vi "Query Instrument Version.vi"(0 "VISA resource name":refnum<visa-resource-name>, 5 "FPGA (0:Hardware Controller FPGA on Main Unit)":i32(ring) items=["Hardware Controller FPGA on Main Unit", "Control PLD And Panel on Main Unit", "Measure PCI FPGA on Main Unit", "Measure Core FPGA on Main Unit", "Measure COM DSP on Main Unit", "RF FPGA on SA RF Unit", "RF FPGA on SA 13GHz RF Unit", "Baseband FPGA on VSG Unit", "RF FPGA on VSG Unit", "Down Conv FPGA on Down Convertor Unit", "2nd Conv FPGA on 2nd Convertor Unit", "ATT_Driver FPGA on ATT Driver Unit", "Hardware Controller FPGA", "Control PLD And Panel", "IF/Local FPGA", "RF/Micro FPGA", "PCI FPGA on Measure Unit", "Core FPGA on Measure Unit", "COM DSP on Measure Unit", "Core FPGA on Measure Option Unit", "Baseband FPGA on SG Unit", "RF FPGA on SG Unit", "BBIF Interface FPGA", "BBIF Main FPGA", "BBIF PCI FPGA", "All FPGA"], 7 "Application (0:Signal Analyzer)":i32(ring) items=["Signal Analyzer", "Spectrum Analyzer", "Phase Noise", "Power Meter", "BER Test"], 9 "Hardware (0:Main Unit)":i32(ring) items=["Main Unit", "SA RF Unit", "SA 13GHz RF Unit", "VSG Unit", "Down Converter Unit", "2nd Converter Unit", "ATT_Driver Unit", "Revision number", "IF Unit", "IF/Local Unit", "RF/Micro Unit", "Measure Unit", "Measure Option Unit", "SG Unit", "CPU Unit", "BBIF Unit", "All"], 11 "error in (no error)":errorcluster) -> (4 "VISA resource name out":refnum<visa-resource-name>, 6 "FPGA Version Number":string, 8 "SW Version Number":string, 10 "HW Revision Number":string, 15 "error out":errorcluster)   [LabVIEW 2020, in "Anritsu Signal Analyzer Series.lvlib"]
doc: "Queries the instrument version(software, hardware and FPGA)."
uses:
  Anritsu Signal Analyzer Series.lvlib
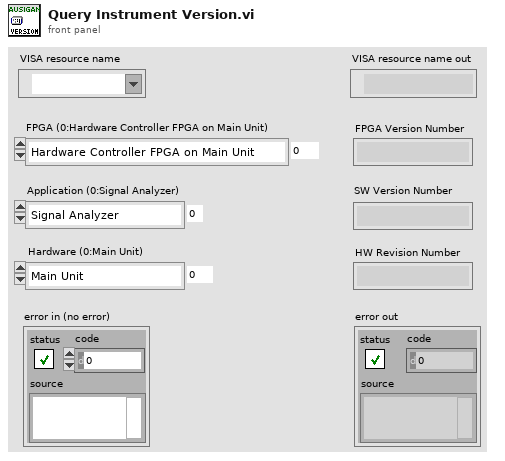
[diagram p1: front panel]
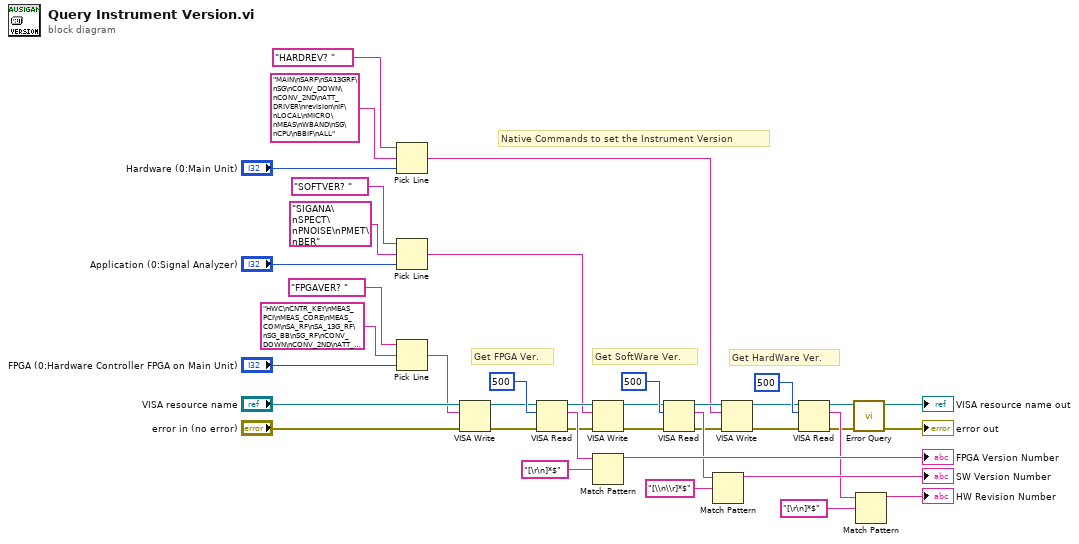
[diagram p0: block diagram]
diagram:
  # "Native Commands to set the Instrument Version"
  # "Get HardWare Ver."
  # "Get SoftWare Ver."
  # "Get FPGA Ver."
  n1 = Pick Line(string ("")="HARDREV? " ("_Command"), multi-line string="MAIN\nSARF\nSA13GRF\nSG\nCONV_DOWN\nCONV_2ND\nATT_DRIVER\nrevision\nIF\nLOCAL\nMICRO\nMEAS\nWBAND\nSG\nCPU\nBBIF\nALL" ("文字列"), line index="Hardware (0:Main Unit)") -> (output string=w10:string)
  n2 = Pick Line(string ("")="SOFTVER? " ("_Command"), multi-line string="SIGANA\nSPECT\nPNOISE\nPMET\nBER" ("文字列"), line index="Application (0:Signal Analyzer)") -> (output string=w9:string)
  n3 = Pick Line(string ("")="FPGAVER? " ("_Command"), multi-line string="HWC\nCNTR_KEY\nMEAS_PCI\nMEAS_CORE\nMEAS_COM\nSA_RF\nSA_13G_RF\nSG_BB\nSG_RF\nCONV_DOWN\nCONV_2ND\nATT_DRIVER\nHWC\nCNTR_KEY\nLOCAL\nMICRO\nMEAS_PCI\nMEAS_CORE\nMEAS_COM\nMEAS_HS_CORE\nSGBB\nSGRF\nBBIFIF\nBBIFMAIN\nBBIFPCI\nALL" ("String"), line index="FPGA (0:Hardware Controller FPGA on Main Unit)") -> (output string=w4:string)
  n4 = VISA Write(VISA resource name="VISA resource name", write buffer=w4, error in (no error)="error in (no error)") -> (VISA resource name out=w29:refnum<visa-resource-name>, error out=w30:errorcluster)  [unwired: 1 out]
  n5 = VISA Read(VISA resource name=w29, byte count=u32 500 ("byte count (0)"), error in (no error)=w30) -> (VISA resource name out=w24:refnum<visa-resource-name>, read buffer=w33:string, error out=w23:errorcluster)  [unwired: 1 out]
  n6 = VISA Write(VISA resource name=w24, write buffer=w9, error in (no error)=w23) -> (VISA resource name out=w25:refnum<visa-resource-name>, error out=w22:errorcluster)  [unwired: 1 out]
  n7 = Match Pattern(string=w33, regular expression="[\r\n]*$" ("search string")) -> (before substring=→"FPGA Version Number":string)  [unwired: 1 in, 3 out]
  n8 = VISA Read(VISA resource name=w25, byte count=u32 500 ("byte count (0)"), error in (no error)=w22) -> (VISA resource name out=w16:refnum<visa-resource-name>, read buffer=w28:string, error out=w2:errorcluster)  [unwired: 1 out]
  n9 = Match Pattern(string=w28, regular expression="[\\n\\r]*$") -> (before substring=→"SW Version Number":string)  [unwired: 1 in, 3 out]
  n10 = VISA Write(VISA resource name=w16, write buffer=w10, error in (no error)=w2) -> (VISA resource name out=w17:refnum<visa-resource-name>, error out=w18:errorcluster)  [unwired: 1 out]
  n11 = VISA Read(VISA resource name=w17, byte count=u32 500 ("byte count (0)"), error in (no error)=w18) -> (VISA resource name out=w15:refnum<visa-resource-name>, read buffer=w21:string, error out=w14:errorcluster)  [unwired: 1 out]
  n12 = call "Error Query.vi"("error in (no error)"=w14, "VISA resource name"=w15) -> ("error out"=→"error out":errorcluster, "VISA resource name out"=→"VISA resource name out":refnum<visa-resource-name>)  [unwired: 6 in, 2 out]
  n13 = Match Pattern(string=w21, regular expression="[\r\n]*$" ("search string")) -> (before substring=→"HW Revision Number":string)  [unwired: 1 in, 3 out]
